vi "Set Master RIO.vi"(8 "error in (no error)":errorcluster, 10 "RIO Device Address":string, 11 "EST Custom Device in":refnum<k24>) -> (0 "error out":errorcluster, 3 "EST Custom Device out":refnum<k24>)   [LabVIEW 2017, in "Engine Simulation Toolkit Scripting API.lvlib"]
uses:
  Engine Simulation Toolkit Scripting API.lvlib
  NationalInstruments.VeriStand.SystemDefinitionAPI
  Shared/Properties.vi
  <vilib>/NI Veristand/Custom Device API/Set Item Property (String).vi
  Shared/Engine Simulation Toolkit Shared.lvlib
  <vilib>/NI Veristand/Custom Device API/Custom Device API.lvlib
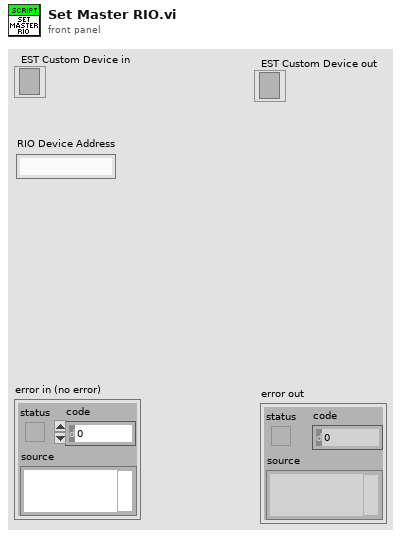
[diagram p1: front panel]
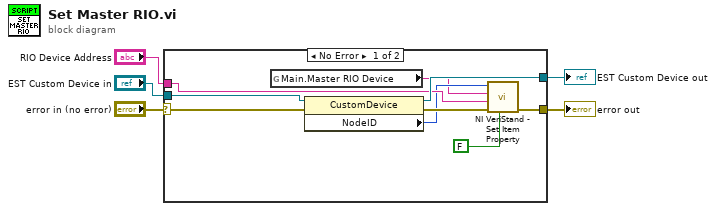
[diagram p0: block diagram]
diagram:
  n1 = case shown="No Error" "error in (no error)" {
    selector: "error in (no error)" -> [w13 w16]
    tunnel: [w10 w16] -> w5
    tunnel: "EST Custom Device in" -> [w14 w15]
    tunnel: [w12 w15] -> w2
    tunnel: "RIO Device Address" -> [w11 _]
    frame No Error {
      n2 = global read "Properties.vi" "Main.Master RIO Device"() -> (w7:string)
      n3 = property class="CustomDevice"(reference=w14, error in=w13) -> (reference out=w12:refnum<k24>, error out=w9:errorcluster, "NodeID"=w8:u64)
      n4 = call-poly <vilib>:"NI VeriStand - Set Item Property.vi"("Binary String (T)"=FALSE, "error in (no error)"=w9, "Value"=w11, "Property Name"=w7, "Item Ref in"=w8) -> ("error out"=w10:errorcluster)  [unwired: 4 in, 2 out]
    }
    frame Error {
    }
  }
  "EST Custom Device out" <- w2
  "error out" <- w5
